vi "go_to_next_line_backup.vi"(8 "error in (no error)":errorcluster, 10 "Message_command in":T2={"No. of command"=3, "Parameters"=["2.31", "s"], "Address"="", "Boolean"=TRUE, "No. of line"=3, "Initial Time"=timestamp(3642518447.490892 s since 1904-01-01), "Current Time"=timestamp(0 s since 1904-01-01), "Status"="Stop DAQ...", "Sequence Ref."=refnum, "Temp check"=0, "Sequence_History"="", "Subsequence"=[]}, 11 "Command Queue in":T1) -> (0 "error out":errorcluster, 3 "Command Queue out":T1)   [LabVIEW 2021]
uses:
  Command_Message.ctl
  Command_Queue.ctl
panel:
  out "concatenated string":string="2:40 PM\tStop DAQ..."
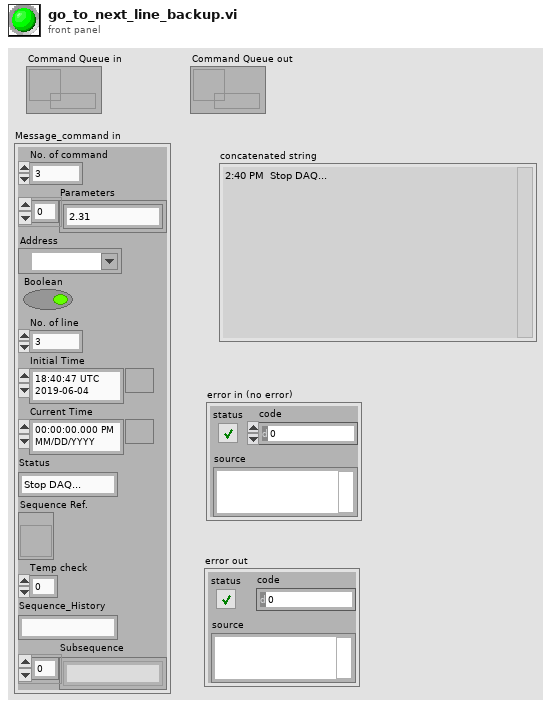
[diagram p1: front panel]
types:
  T1 = typedef "Command_Queue.ctl" = refnum<queue>
  T2 = typedef "Command_Message.ctl" = cluster{"No. of command":i32, "Parameters":string[], "Address":refnum<visa-resource-name>, "Boolean":bool, "No. of line":i32, "Initial Time":timestamp, "Current Time":timestamp, "Status":string, "Sequence Ref.":refnum<vi>, "Temp check":i32, "Sequence_History":string, "Subsequence":string[]}
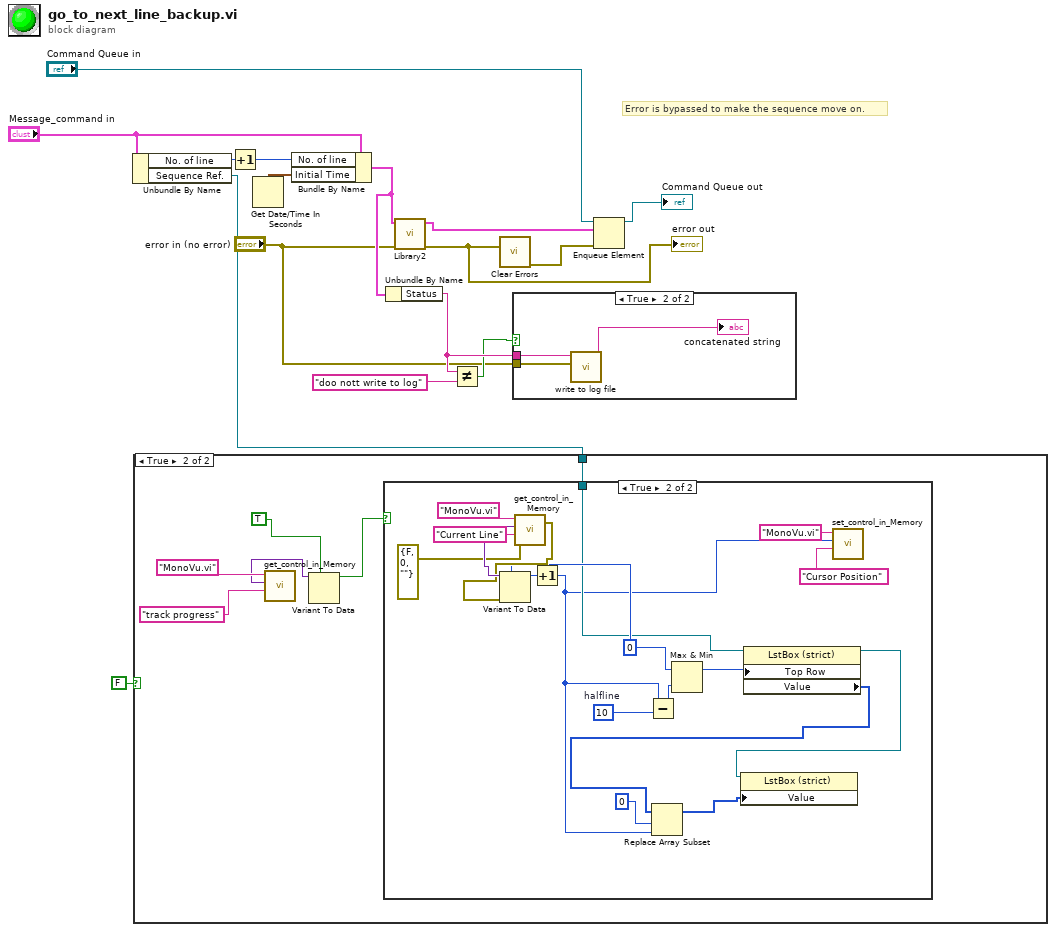
[diagram p0: block diagram]
diagram:
  # "Error is bypassed to make the sequence move on."
  n1 = Unbundle By Name("Message_command in") -> ("No. of line"=w12:i32, "Sequence Ref."=w2:refnum<vi>)
  n2 = case shown="True" FALSE {
    tunnel: w2 -> [_ w17]
    frame False {
    }
    frame True {
      n3 = call "get_control_in_Memory.vi"("Control Name"="track progress", "VI Name"="MonoVu.vi") -> ("Value"=w20:variant)  [unwired: 2 in, 1 out]
      n4 = Variant To Data(type=TRUE ("track progress"), Variant=w20) -> (data=w18:bool)  [unwired: 1 in, 1 out]
      n5 = case shown="True" w18 {
        tunnel: w17 -> [_ w26]
        frame False {
        }
        frame True {
          w28 = u8 0 ("x")
          w30 = 10  # halfline
          n6 = call "get_control_in_Memory.vi"("error in (no error)"=errorcluster {"status"=FALSE, "code"=0, "source"=""}, "Control Name"="Current Line", "VI Name"="MonoVu.vi") -> ("error out 2"=w36:errorcluster, "Value"=w39:variant)  [unwired: 1 in]
          n7 = Variant To Data(error in=w36, type=w28, Variant=w39) -> (data=w27:u8)  [unwired: 1 out]
          n8 = Increment(x=w27) -> (x+1=w23:u8)
          n9 = Subtract(x=w23, y=w30) -> (x-y=w32:i32)
          n10 = Max & Min(x=w28, y=w32) -> (max(x,y)=w31:i32)  [unwired: 1 out]
          n11 = property on="Property Node" class="LstBox (strict)"(reference=w26, "Top Row"=w31) -> (reference out=w34:refnum<vi>, "Value"=w33:i32[])  [unwired: 1 in, 1 out]
          n12 = Replace Array Subset(array=w33, new element=w23, index=0) -> (w35:i32[])
          n13 = property on="Property Node" class="LstBox (strict)"(reference=w34, "Value"=w35) -> ()  [unwired: 1 in, 2 out]
          n14 = call "set_control_in_Memory.vi"("Control Name"="Cursor Position", "Value"=w23, "VI Name"="MonoVu.vi") -> ()  [unwired: 2 in, 1 out]
        }
      }
    }
  }
  n15 = Increment(x=w12) -> (x+1=w15:i32)
  n16 = Get Date/Time In Seconds() -> (seconds since 1Jan1904=w16:timestamp)
  n17 = Bundle By Name(cluster="Message_command in", "No. of line"=w15, "Initial Time"=w16) -> (w9:T2)
  n18 = Unbundle By Name(w9) -> ("Status"=w8:string)
  n19 = call "Library2.vi"("Message_command_in"=w9, "error in (no error)"="error in (no error)") -> ("Message_command out"=w10:T2, "error out"=w3:errorcluster)  [unwired: 7 in]
  "error out" <- w3
  n20 = Not Equal?(x=w8, y="doo nott write to log") -> (x != y?=w6:bool)
  n21 = call <vilib>:"Clear Errors.vi"("error in (no error)"=w3) -> ("error out"=w4:errorcluster)  [unwired: 5 in, 1 out]
  n22 = case shown="True" w6 {
    tunnel: w8 -> [_ w43]
    tunnel: "error in (no error)" -> [_ w41]
    frame False {
    }
    frame True {
      n23 = call "write to log file.vi"("input"=w43, "error in"=w41) -> ("log"=→"concatenated string":string)  [unwired: 8 in]
    }
  }
  n24 = Enqueue Element(queue="Command Queue in", element=w10, error in (no error)=w4) -> (queue out=→"Command Queue out":T1)  [unwired: 1 in, 2 out]
